vi "controlAQuadBOutClock.vi"(7 "Set":bool, 8 "error in":errorcluster, 9 "clock in":i32, 10 "axis in":u8, 11 "connection ID":refnum<k5>) -> (0 "error out":errorcluster, 1 "clock out":i32, 2 "axis out":u8, 3 "connection ID":refnum<k5>)   [LabVIEW 2016]
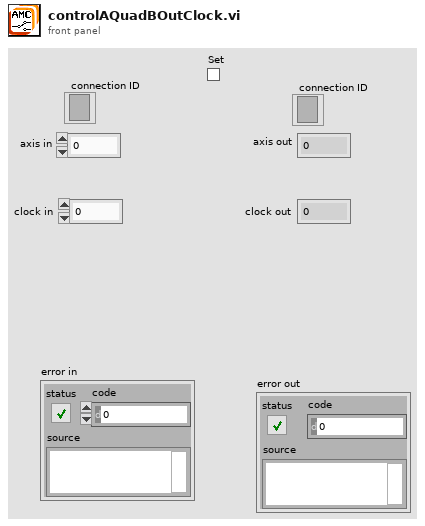
[diagram p1: front panel]
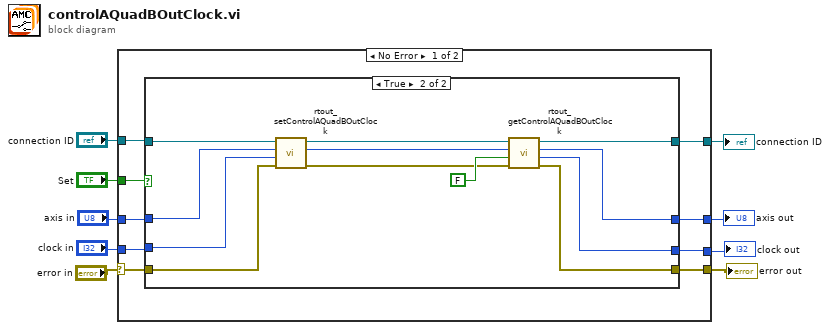
[diagram p0: block diagram]
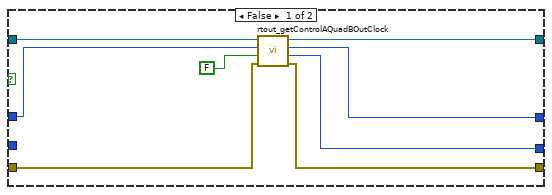
[diagram p2: hidden frame]
diagram:
  n1 = case shown="No Error" "error in" {
    selector: "error in" -> [w10 w41]
    tunnel: "axis in" -> [w16 w40]
    tunnel: [w11 w41] -> w8
    tunnel: [w15 w40] -> w7
    tunnel: "Set" -> [w14 _]
    tunnel: [w17 w39] -> w5
    tunnel: "connection ID" -> [w18 w39]
    tunnel: "clock in" -> [w12 w42]
    tunnel: [w13 w42] -> w2
    frame No Error {
      n2 = case shown="True" w14 {
        tunnel: [w24 w32] -> w17
        tunnel: w18 -> [w25 w38]
        tunnel: w16 -> [w26 w36]
        tunnel: [w20 w29] -> w15
        tunnel: [w21 w30] -> w13
        tunnel: [w22 w31] -> w11
        tunnel: w12 -> [_ w35]
        tunnel: w10 -> [w23 w37]
        frame False {
          n3 = call "rtout_getControlAQuadBOutClock.vi"("error in"=w23, "tempvalue"=FALSE, "axis"=w26, "connection ID"=w25) -> ("error out"=w22:errorcluster, "clock_in_ns"=w21:i32, "axis_out"=w20:i32, "connection ID"=w24:refnum<k5>)  [unwired: 4 in]
        }
        frame True {
          n4 = call "rtout_setControlAQuadBOutClock.vi"("error in"=w37, "clock"=w35, "axis"=w36, "connection ID"=w38) -> ("error out"=w27:errorcluster, "axis_out"=w28:i32, "connection ID"=w33:refnum<k5>)  [unwired: 5 in]
          n5 = call "rtout_getControlAQuadBOutClock.vi"("error in"=w27, "tempvalue"=FALSE, "axis"=w28, "connection ID"=w33) -> ("error out"=w31:errorcluster, "clock_in_ns"=w30:i32, "axis_out"=w29:i32, "connection ID"=w32:refnum<k5>)  [unwired: 4 in]
        }
      }
    }
    frame Error {
    }
  }
  "error out" <- w8
  "axis out" <- w7
  "connection ID" <- w5
  "clock out" <- w2
